vi "ClassPanel.vi"(8 "error in (no error)":errorcluster caption="entrée d'erreur (pas d'erreur)", 11 "LSCI332.lvclass":refnum<class "LSCI332.lvclass">) -> (0 "error out":errorcluster caption="sortie d'erreur", 3 "LSCI332.lvclass Out":refnum<class "LSCI332.lvclass">)   [LabVIEW 2019, in "LSCI332.lvclass"]
uses:
  LSCI332.lvclass
  C:/Programmes Labview/LabScanV1A/DevicesClass/BaseDevice/BaseDevice.lvclass
  BaseDevice/Accessor/GetClassEvent.vi
panel:
  in  "MainProgQEvent":refnum<user-event>
  in  "MainProgQ":refnum<queue>
  in  "Acq":bool
  out "Résistance":u16=50 caption="Résistance Chauffage"
  in  "Boucle(1)":u32(ring) caption="Boucle" items=["Boucle 1", "Boucle 2"]
  out "SensorA":dbl=60.0 caption="Sensor A (U)" min=0.1 step=0.1 format="%#.3f"
  out "P(%)":dbl caption="Power(%)"
  out "SensorB":dbl=60.0 caption="Sensor B (U)" min=0.1 step=0.1 format="%#.3f"
  out "TempB":dbl=60.0 caption="Temp B (K)" min=0.1 step=0.1 format="%#.3f"
  in  "SetPoint":dbl=293.0 caption="Setpoint" min=0.005 max=500.0 step=0.001 format="%#.3g"
  in  "ManOutput":dbl caption="Man Output %" format="%#.2g"
  in  "HtrRange":u16(ring) caption="Heat Scale" items=["Off", "Low (.5W)", "Med (5W)", "High (50W)"]
  in  "Stop":bool
  in  "MiseAJour":bool
  out "TempA":dbl=60.0 caption="Temp A (K)" min=0.1 step=0.1 format="%#.3f"
  out "Init Program":bool
  # "this MUST labeled with class name"
  # "this MUST be present and labeled \"Stop\""
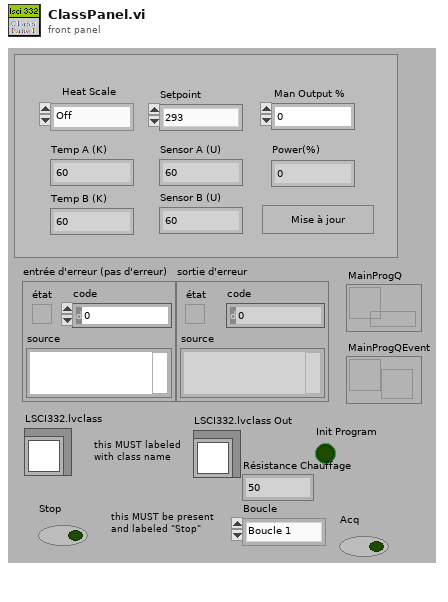
[diagram p1: front panel]
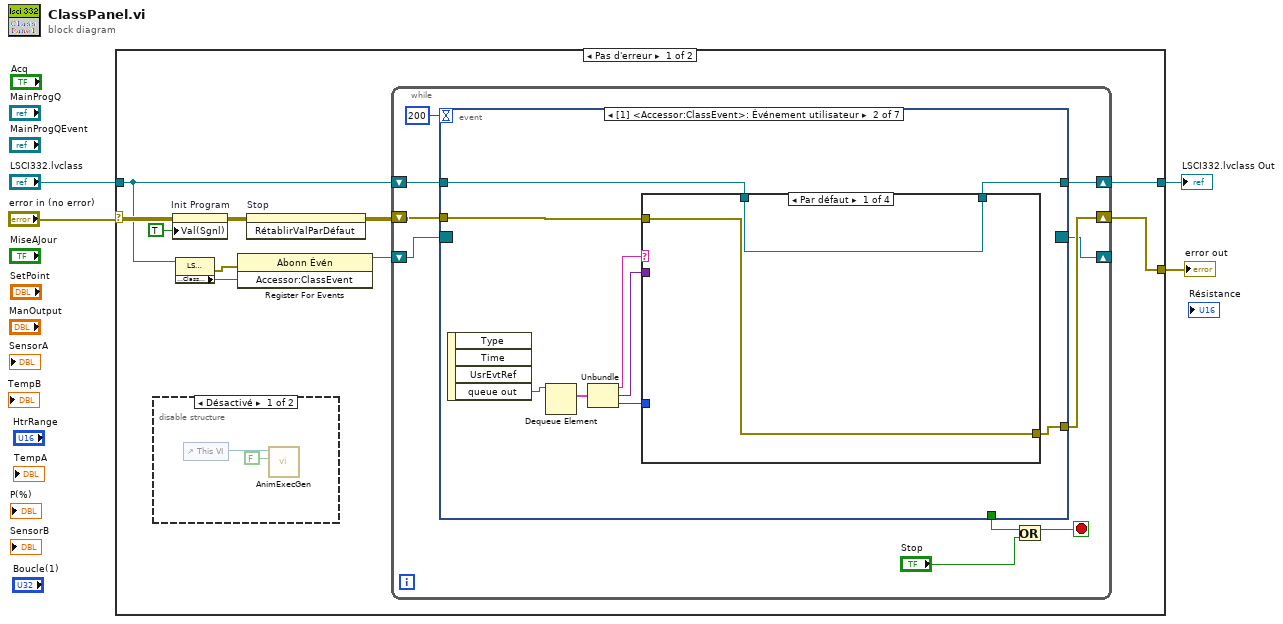
[diagram p0: block diagram]
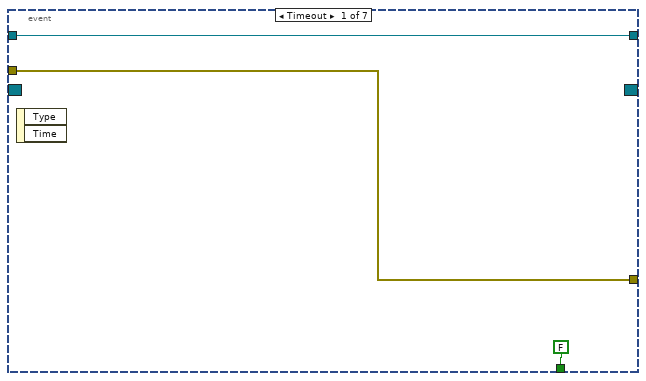
[diagram p3: hidden frame]
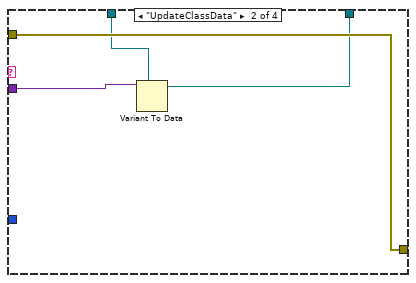
[diagram p4: hidden frame]
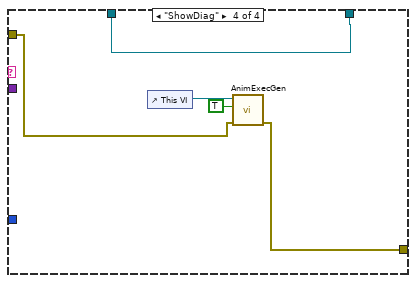
[diagram p6: hidden frame]
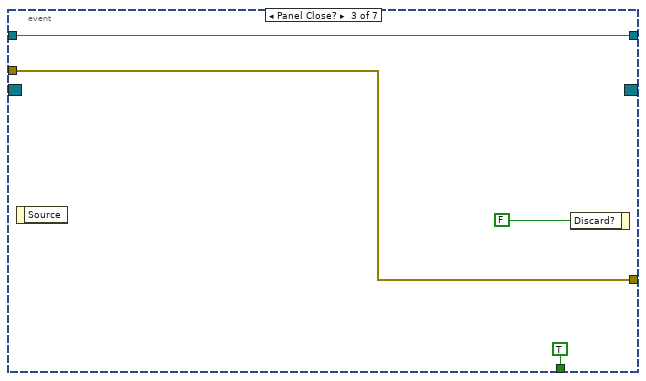
[diagram p7: hidden frame]
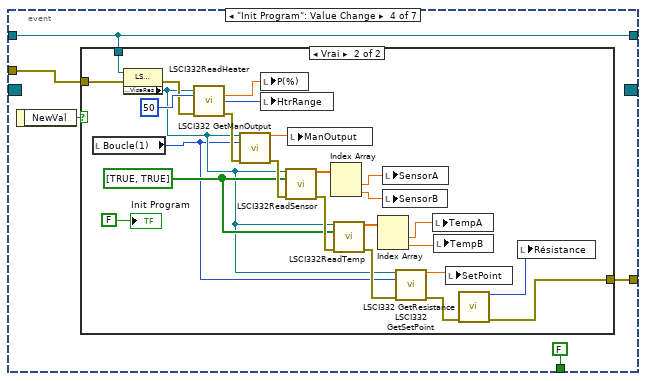
[diagram p8: hidden frame]
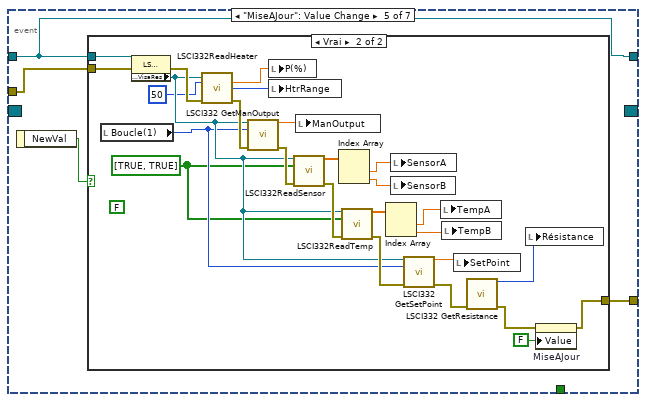
[diagram p10: hidden frame]
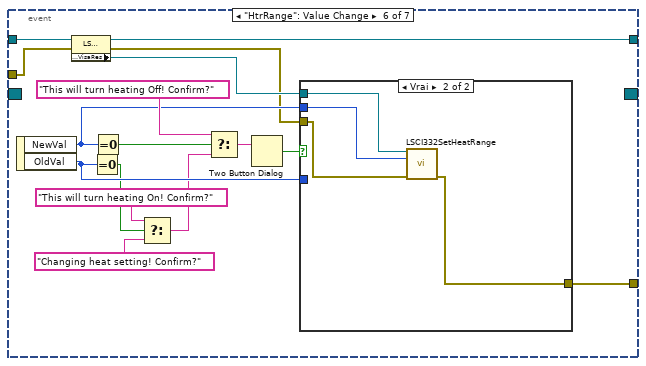
[diagram p12: hidden frame]
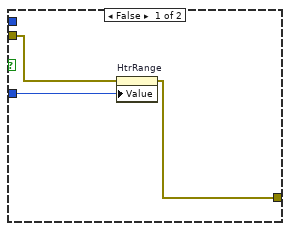
[diagram p13: hidden frame]
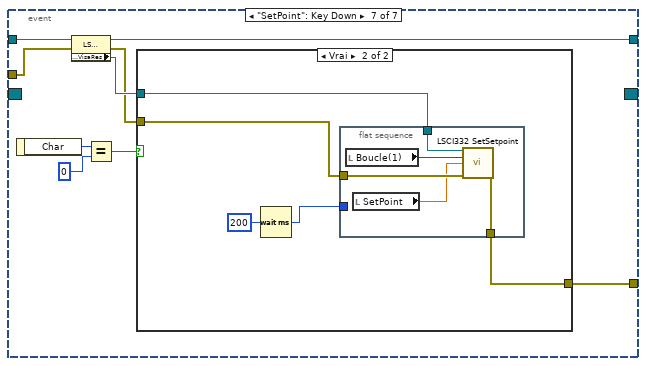
[diagram p14: hidden frame]
diagram:
  n1 = case shown="Pas d'erreur" "error in (no error)" {
    selector: "error in (no error)" -> [w11 w162]
    tunnel: [w14 w162] -> w3
    tunnel: "LSCI332.lvclass" -> [w6 w161]
    tunnel: [w12 w161] -> w1
    frame No Error {
      n2 = disable-structure shown="Désactivé" {
        frame Disabled {
          n3 = control-ref of="This VI"() -> (w15:refnum<vi>)
          n4 = call <userlib>:"AnimExecGen.vi"("Animer l'exécution ?"=FALSE, "ViRef"=w15) -> ()  [unwired: 9 in, 1 out]
        }
        frame Enabled {
        }
      }
      n5 = property on="Init Program" class="Bool (strict)"(error in=w11, "Val(Sgnl)"=TRUE ("Valeur (Signalisation)")) -> (error out=w10:errorcluster)  [unwired: 1 in, 1 out]
      n6 = property class="LSCI332.lvclass"(reference=w6) -> (error out=w8:errorcluster, "Accessor:ClassEvent"=w7:refnum<user-event>)  [unwired: 1 in, 1 out]
      n7 = register-events(error in=w8, w7) -> (reference out=w5:refnum<event-registration>)  [unwired: 1 in, 1 out]
      n8 = invoke on="Stop" class="Bool (strict)" method="RétablirValParDéfaut"(error in=w10) -> (error out=w9:errorcluster)  [unwired: 2 in, 2 out]
      n9 = while {
        shift-right: [w24] -> w14
        shift-left: w9 -> [w25]
        shift-right: [w21] -> w12
        shift-left: w6 -> [w23]
        shift-right: [w17] -> _
        shift-left: w5 -> [w18]
        stop <- w20 stop-if-true
        n10 = event shown="[1] <Accessor:ClassEvent>: Événement utilisateur" {
          selector: w18 -> [_ _ _ _ _ _ _]
          dyn-events: [_ _ _ _ _ _ _] -> w17
          timeout: 200 -> [_ _ _ _ _ _ _]
          tunnel: w25 -> [w27 w37 w53 w59 w87 w121 w147]
          tunnel: [w27 w31 w53 w58 w89 w118 w144] -> w24
          tunnel: w23 -> [w28 w38 w52 w56 w88 w123 w149]
          tunnel: [FALSE _ TRUE FALSE _ _ _] -> w22
          tunnel: [w28 w30 w52 w56 w88 w122 w148] -> w21
          event Timeout {
            n11 = event-data() -> ()  [unwired: 1 in, 2 out]
          }
          event User Event {
            n12 = event-data() -> ("queue out"=w35:refnum<queue>)  [unwired: 1 in, 3 out]
            n13 = Dequeue Element(queue=w35) -> (element=w36:cluster{"Message":string, "Data":variant, i32})  [unwired: 2 in, 3 out]
            n14 = Unbundle(w36) -> ("Message"=w34:string, "Data"=w33:variant, w32:i32)
            n15 = case shown="Par défaut" w34 {
              tunnel: w37 -> [w40 w44 w45 w49]
              tunnel: w33 -> [_ w43 _ _]
              tunnel: w38 -> [w39 w42 w46 w47]
              tunnel: [w39 w41 w46 w47] -> w30
              tunnel: [w40 w44 w45 w48] -> w31
              tunnel: w32 -> [_ _ _ _]
              frame Default {
              }
              frame "UpdateClassData" {
                n16 = Variant To Data(type=w42, Variant=w43) -> (data=w41:refnum<class "LSCI332.lvclass">)  [unwired: 1 in, 1 out]
              }
              frame "MeasDone" {
              }
              frame "ShowDiag" {
                n17 = control-ref of="This VI"() -> (w50:refnum<vi>)
                n18 = call <userlib>:"AnimExecGen.vi"("ErrorIn(No Error)"=w49, "Animer l'exécution ?"=TRUE, "ViRef"=w50) -> ("sortie d'erreur"=w48:errorcluster)  [unwired: 8 in]
              }
            }
          }
          event Panel Close? {
            n19 = event-data() -> ()  [unwired: 1 in, 1 out]
            n20 = event-data("Discard?"=FALSE ("Rejeter ?")) -> ()  [unwired: 1 in, 1 out]
          }
          event "Init Program": Value Change {
            n21 = event-data() -> ("NewVal"=w60:bool)  [unwired: 1 in]
            n22 = case shown="Vrai" w60 {
              tunnel: w59 -> [w61 w84]
              tunnel: [w61 w63] -> w58
              tunnel: w56 -> [_ w85]
              frame False {
              }
              frame True {
                w72 = bool[] [TRUE, TRUE] ("Activées")
                n23 = local read "Boucle(1)"() -> (w64:u32)
                n24 = property class="LSCI332.lvclass"(reference=w85, error in=w84) -> (error out=w82:errorcluster, "Accessor:VisaRes"=w67:refnum<visa-resource-name>)  [unwired: 1 out]
                n25 = call <userlib>:"LSCI332ReadHeater.vi"("VISA Rsrc"=w67, "Résistance"=u16 50, "error in"=w82) -> ("Puissance(%)"=w81:dbl, "Échelle"=w80:u16, "error out"=w79:errorcluster)  [unwired: 9 in, 1 out]
                n26 = call <userlib>:"LSCI332 GetManOutput.vi"("VISA Rsrc"=w67, "Boucle(1)"=w64, "error in"=w79) -> ("ManOutput"=w78:dbl, "error out"=w77:errorcluster)  [unwired: 11 in]
                n27 = local write "P(%)"(w81) -> ()
                n28 = local write "HtrRange"(w80) -> ()
                n29 = call <userlib>:"LSCI332ReadSensor.vi"("VISA Rsrc"=w67, "Activées"=w72, "error in"=w77) -> ("Données"=w76:dbl[], "error out"=w73:errorcluster)  [unwired: 11 in]
                n30 = local write "ManOutput"(w78) -> ()
                n31 = Index Array(array=w76) -> (element #1=w74:dbl, element #2=w75:dbl)  [unwired: 2 in]
                n32 = call <userlib>:"LSCI332ReadTemp.vi"("VISA Rsrc"=w67, "Activées"=w72, "error in"=w73) -> ("Données"=w71:dbl[], "error out"=w68:errorcluster)  [unwired: 11 in]
                n33 = Index Array(array=w71) -> (element #1=w69:dbl, element #2=w70:dbl)  [unwired: 2 in]
                n34 = local write "SensorA"(w74) -> ()
                n35 = local write "SensorB"(w75) -> ()
                n36 = call <userlib>:"LSCI332 GetSetPoint.vi"("VISA Rsrc"=w67, "Boucle(1)"=w64, "error in (no error)"=w68) -> ("SetPoint"=w66:dbl, "error out"=w65:errorcluster)  [unwired: 11 in]
                n37 = local write "TempA"(w69) -> ()
                n38 = local write "TempB"(w70) -> ()
                n39 = local write "SetPoint"(w66) -> ()
                n40 = call <userlib>:"LSCI332 GetResistance.vi"("error in"=w65) -> ("Résistance"=w62:u16, "error out"=w63:errorcluster)  [unwired: 13 in]
                n41 = local write "Résistance"(w62) -> ()
                "Init Program" <- FALSE
              }
            }
          }
          event "MiseAJour": Value Change {
            n42 = event-data() -> ("NewVal"=w90:bool)  [unwired: 1 in]
            n43 = case shown="Vrai" w90 {
              tunnel: [w91 w94] -> w89
              tunnel: w88 -> [_ w93]
              tunnel: w87 -> [w91 w92]
              frame False {
              }
              frame True {
                w97 = bool[] [TRUE, TRUE] ("Activées")
                (unwired) FALSE
                n44 = local read "Boucle(1)"() -> (w99:u32)
                n45 = property class="LSCI332.lvclass"(reference=w93, error in=w92) -> (error out=w116:errorcluster, "Accessor:VisaRes"=w102:refnum<visa-resource-name>)  [unwired: 1 out]
                n46 = call <userlib>:"LSCI332ReadHeater.vi"("VISA Rsrc"=w102, "Résistance"=u16 50, "error in"=w116) -> ("Puissance(%)"=w115:dbl, "Échelle"=w114:u16, "error out"=w113:errorcluster)  [unwired: 9 in, 1 out]
                n47 = call <userlib>:"LSCI332 GetManOutput.vi"("VISA Rsrc"=w102, "Boucle(1)"=w99, "error in"=w113) -> ("ManOutput"=w112:dbl, "error out"=w111:errorcluster)  [unwired: 11 in]
                n48 = local write "P(%)"(w115) -> ()
                n49 = local write "HtrRange"(w114) -> ()
                n50 = call <userlib>:"LSCI332ReadSensor.vi"("VISA Rsrc"=w102, "Activées"=w97, "error in"=w111) -> ("Données"=w110:dbl[], "error out"=w107:errorcluster)  [unwired: 11 in]
                n51 = local write "ManOutput"(w112) -> ()
                n52 = Index Array(array=w110) -> (element #1=w108:dbl, element #2=w109:dbl)  [unwired: 2 in]
                n53 = call <userlib>:"LSCI332ReadTemp.vi"("VISA Rsrc"=w102, "Activées"=w97, "error in"=w107) -> ("Données"=w106:dbl[], "error out"=w103:errorcluster)  [unwired: 11 in]
                n54 = Index Array(array=w106) -> (element #1=w104:dbl, element #2=w105:dbl)  [unwired: 2 in]
                n55 = local write "SensorA"(w108) -> ()
                n56 = local write "SensorB"(w109) -> ()
                n57 = call <userlib>:"LSCI332 GetSetPoint.vi"("VISA Rsrc"=w102, "Boucle(1)"=w99, "error in (no error)"=w103) -> ("SetPoint"=w101:dbl, "error out"=w100:errorcluster)  [unwired: 11 in]
                n58 = local write "TempA"(w104) -> ()
                n59 = local write "TempB"(w105) -> ()
                n60 = local write "SetPoint"(w101) -> ()
                n61 = call <userlib>:"LSCI332 GetResistance.vi"("error in"=w100) -> ("Résistance"=w98:u16, "error out"=w95:errorcluster)  [unwired: 13 in]
                n62 = local write "Résistance"(w98) -> ()
                n63 = property on="MiseAJour" class="Bool (strict)"(error in=w95, "Value"=FALSE ("MiseAJour")) -> (error out=w94:errorcluster)  [unwired: 1 in, 1 out]
              }
            }
          }
          event "HtrRange": Value Change {
            n64 = event-data() -> ("NewVal"=w129:u16, "OldVal"=w128:u16)  [unwired: 1 in]
            n65 = property class="LSCI332.lvclass"(reference=w123, error in=w121) -> (reference out=w122:refnum<class "LSCI332.lvclass">, error out=w119:errorcluster, "Accessor:VisaRes"=w120:refnum<visa-resource-name>)
            n66 = Equal To 0?(x=w128) -> (x = 0?=w127:bool)
            n67 = Equal To 0?(x=w129) -> (x = 0?=w133:bool)
            n68 = Select(t="This will turn heating On! Confirm?", s=w127, f="Changing heat setting! Confirm?") -> (s? t:f=w124:string)
            n69 = Select(t="This will turn heating Off! Confirm?", s=w133, f=w124) -> (s? t:f=w131:string)
            n70 = Two Button Dialog(message=w131) -> (T button?=w130:bool)  [unwired: 2 in]
            n71 = case shown="Vrai" w130 {
              tunnel: w128 -> [w136 _]
              tunnel: w129 -> [_ w139]
              tunnel: w120 -> [_ w140]
              tunnel: w119 -> [w135 w138]
              tunnel: [w134 w137] -> w118
              frame False {
                n72 = property on="HtrRange" class="MDér (strict)"(error in=w135, "Value"=w136) -> (error out=w134:errorcluster)  [unwired: 1 in, 1 out]
              }
              frame True {
                n73 = call <userlib>:"LSCI332SetHeatRange.vi"("VISA Rsrc"=w140, "HtrRange"=w139, "error in"=w138) -> ("error out"=w137:errorcluster)  [unwired: 12 in]
              }
            }
          }
          event "SetPoint": Key Down {
            n74 = event-data() -> ("Char"=w142:i16)  [unwired: 1 in]
            n75 = property class="LSCI332.lvclass"(reference=w149, error in=w147) -> (reference out=w148:refnum<class "LSCI332.lvclass">, error out=w145:errorcluster, "Accessor:VisaRes"=w146:refnum<visa-resource-name>)
            n76 = Equal?(x=w142, y=i16 0) -> (x = y?=w141:bool)
            n77 = case shown="Vrai" w141 {
              tunnel: w146 -> [_ w153]
              tunnel: w145 -> [w150 w155]
              tunnel: [w150 w154] -> w144
              frame False {
              }
              frame True {
                n78 = Wait (ms)(milliseconds to wait=u32 200) -> (millisecond timer value=w151:u32)
                n79 = flat-sequence {
                  tunnel: w155 -> [w160]
                  tunnel: [w159] -> w154
                  tunnel: w153 -> [w156]
                  tunnel: w151 -> [_]
                  frame #0 {
                    n80 = local read "Boucle(1)"() -> (w157:u32)
                    n81 = local read "SetPoint"() -> (w158:dbl)
                    n82 = call <userlib>:"LSCI332 SetSetpoint.vi"("VISA Rsrc"=w156, "Boucle(1)"=w157, "SetPoint"=w158, "error in (no error)"=w160) -> ("error out"=w159:errorcluster)  [unwired: 11 in]
                  }
                }
              }
            }
          }
        }
        n83 = Or(x=w22, y="Stop") -> (x .or. y?=w20:bool)
      }
    }
    frame Error {
    }
  }
  "error out" <- w3
  "LSCI332.lvclass Out" <- w1
